vi "add 4200 initalize(SubVI).vi"(9 "字符串":string, 10 "model":string="Delta") -> (0 "连接的字符串":string, 3 "ok or cancel":bool=TRUE)   [LabVIEW 2019, in "initialize.lvlib"]
uses:
  initialize.lvlib
panel:
  in  "SMU2(Ryx) Setup":T1={"Enable"=TRUE, "Source Mode"=enum."Current Source", "Compliance (V/A)"=0.1, "Source V/I (V/A)"=0.0, "Current Measurement Range\n(Limited Auto)"=9} {"Current Measurement Range\n(Limited Auto)" items=["1 pA (pre-Amp only)", "10 pA (pre-Amp only)", "100 pA (pre-Amp only)", "1 nA", "10 nA", "100 nA", "1 uA", "10 uA", "100 uA", "1 mA", "10 mA", "100 mA", "1 A (4210-SMU only)"]; "Source V/I (V/A)" min=-100.0 max=100.0 step=0.0001 format="%^.2e"; "Compliance (V/A)" min=-210.0 max=210.0 format="%_3e"}
  in  "SMU1(Rxx) Setup":T1={"Enable"=TRUE, "Source Mode"=enum."Current Source", "Compliance (V/A)"=0.1, "Source V/I (V/A)"=0.0, "Current Measurement Range\n(Limited Auto)"=9} {"Current Measurement Range\n(Limited Auto)" items=["1 pA (pre-Amp only)", "10 pA (pre-Amp only)", "100 pA (pre-Amp only)", "1 nA", "10 nA", "100 nA", "1 uA", "10 uA", "100 uA", "1 mA", "10 mA", "100 mA", "1 A (4210-SMU only)"]; "Source V/I (V/A)" format="%^.2e"; "Compliance (V/A)" min=-210.0 max=210.0 format="%_3e"}
  in  "Integration Time":i16(slide)=2 min=1 max=3 step=1 scale=1.0..3.0
  in  "Sampling Mode Timing":T2={"Wait Time"=0.0, "Interval"=0.1, "No. of Readings"=5} {"No. of Readings" min=1 max=4097 step=1; "Interval" min=0.0 max=10.0 step=0.001 format="%.2g"; "Wait Time" min=0.0 max=100.0 step=0.1 format="%.3g"}
  out "错误输出":errorcluster
  in  "load":bool
  in  "cancel":bool
  in  "ok":bool
  # "Please make sure KI 4200 is in Normal Mode (under KCON).\nStart KXCI before running this VI."
  # "Hold up start of test (s)"
  # "Time between measurements(s)"
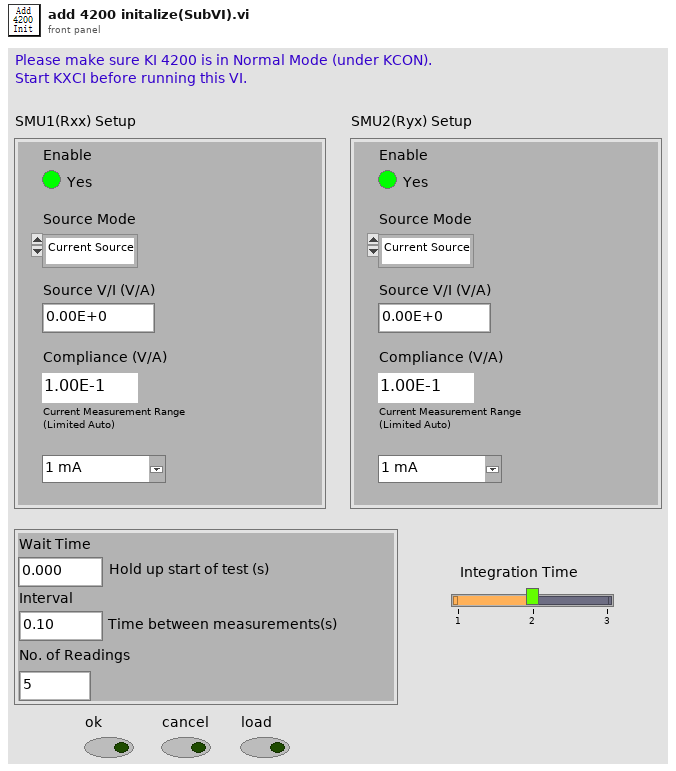
[diagram p1: front panel]
types:
  T1 = cluster{"Enable":bool, "Source Mode":enum16{"Voltage Source", "Current Source", "Common"}, "Compliance (V/A)":dbl, "Source V/I (V/A)":dbl, "Current Measurement Range\n(Limited Auto)":u16}
  T2 = cluster{"Wait Time":dbl, "Interval":dbl, "No. of Readings":i16}
  T3 = enum16{"open", "replace", "create", "open or create", "replace or create"}
  T4 = enum16{"open", "replace", "create", "open or create", "replace or create", "replace or create with confirmation"}
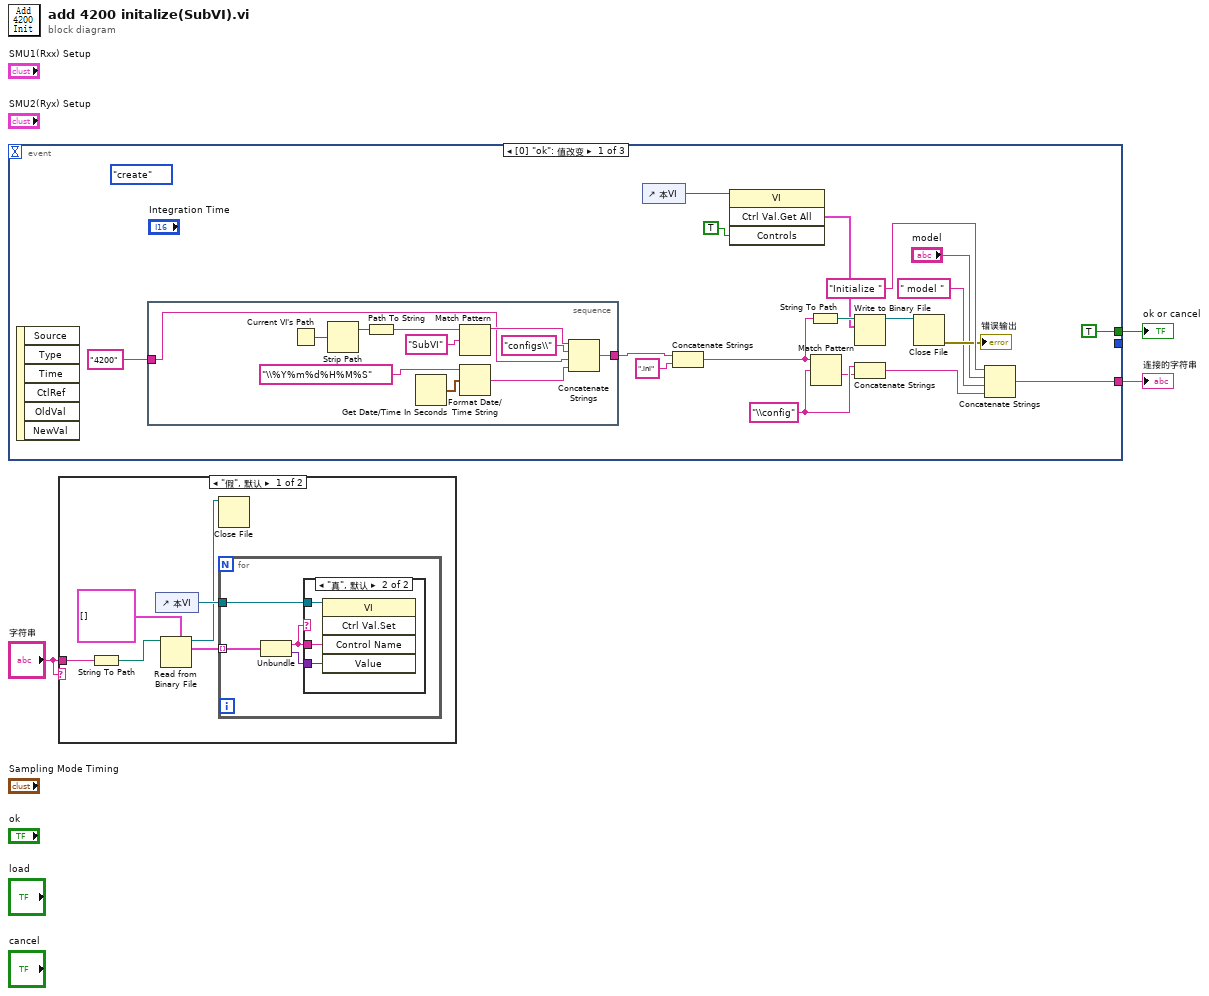
[diagram p0: block diagram]
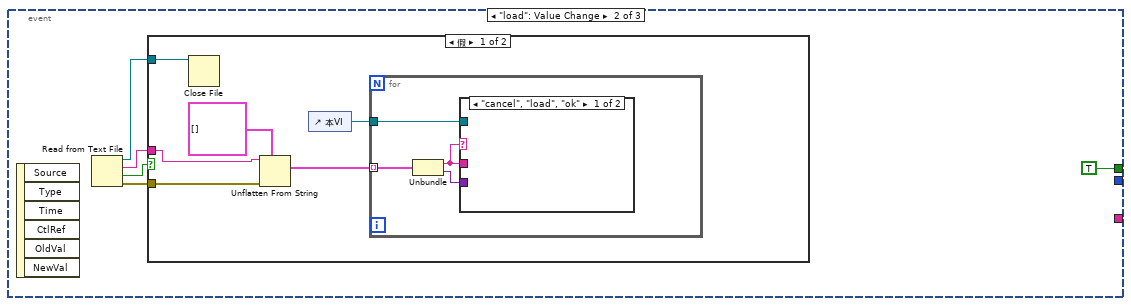
[diagram p4: hidden frame]
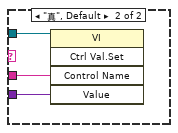
[diagram p5: hidden frame]
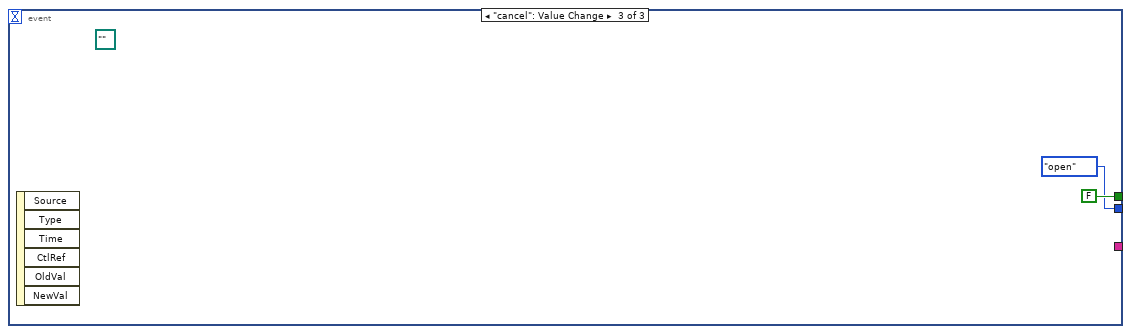
[diagram p7: hidden frame]
diagram:
  n1 = event shown="[0] \"ok\": 值改变" {
    selector: _ -> [_ _ _]
    dyn-events: _ -> [_ _ _]
    timeout: _ -> [_ _ _]
    tunnel: [_ _ T3."open" ("operation(0:open)")] -> _
    tunnel: [TRUE TRUE FALSE] -> w3
    tunnel: [w11 _ _] -> w1
    event "ok": Value Change {
      w7 = "\\config" ("正则表达式")
      (unwired) T4."create" ("操作(0:open)")
      n2 = event-data() -> ()  [unwired: 1 in, 6 out]
      n3 = stacked-sequence {
        tunnel: [w32] -> w16
        tunnel: "4200" ("字符串") -> [w22]
        frame #0 {
          n4 = Current VI's Path() -> (path=w28:path)
          n5 = Strip Path(path=w28) -> (stripped path=w23:path)  [unwired: 1 out]
          n6 = Path To String(path=w23) -> (string=w29:string)
          n7 = Get Date/Time In Seconds() -> (seconds since 1Jan1904=w26:timestamp)
          n8 = Match Pattern(string=w29, regular expression="SubVI" ("正则表达式")) -> (before substring=w31:string)  [unwired: 1 in, 3 out]
          n9 = Format Date/Time String(time format string (%c)="\\%Y%m%d%H%M%S", seconds (now)=w26) -> (date/time string=w27:string)  [unwired: 1 in]
          n10 = Concatenate Strings(w31, "configs\\" ("字符串"), w22, w27) -> (w32:string)
        }
      }
      n11 = control-ref of="本VI"() -> (w19:refnum<vi>)
      n12 = Concatenate Strings(w16, ".ini" ("字符串")) -> (w5:string)
      n13 = invoke class="VI" method="Ctrl Val.Get All"(reference=w19, "Controls"=TRUE ("控件")) -> ("Get All Control Values Variant"=w9:cluster{"Name":string, "Variant Data":variant}[])  [unwired: 2 in, 3 out]
      n14 = String To Path(string=w5) -> (path=w10:path)
      n15 = Match Pattern(string=w5, regular expression=w7) -> (after substring=w6:string)  [unwired: 1 in, 3 out]
      n16 = Write to Binary File(file (use dialog)=w10, data=w9) -> (refnum out=w8:refnum<file>)  [unwired: 4 in, 2 out]
      n17 = Concatenate Strings(w7, w6) -> (w4:string)
      n18 = Close File(refnum=w8) -> (error out=→"错误输出":errorcluster)  [unwired: 1 in, 1 out]
      n19 = Concatenate Strings("Initialize " ("字符串"), "model", " model " ("字符串"), w4) -> (w11:string)
    }
    event "load": Value Change {
      n20 = event-data() -> ()  [unwired: 1 in, 6 out]
      n21 = Read from Text File() -> (refnum out=w36:refnum<file>, text=w34:string, cancelled=w33:bool, error out=w35:errorcluster)  [unwired: 4 in]
      n22 = case shown="假" w33 {
        tunnel: w36 -> [w43 _]
        tunnel: w35 -> [w41 _]
        tunnel: w34 -> [w40 _]
        frame False {
          n23 = Close File(refnum=w43) -> ()  [unwired: 1 in, 2 out]
          n24 = Unflatten From String(type=cluster{"Name":string, "Variant Data":variant}[] [] ("控件值:获取全部"), binary string=w40, error in (no error)=w41) -> (value=w39:cluster{"Name":string, "Variant Data":variant}[])  [unwired: 2 in, 2 out]
          n25 = control-ref of="本VI"() -> (w38:refnum<vi>)
          n26 = for {
            tunnel: w39 -> [w47] mode=indexing
            tunnel: w38 -> [w46]
            n27 = Unbundle(w47) -> ("Name"=w44:string, "Variant Data"=w45:variant)
            n28 = case shown="\"cancel\", \"load\", \"ok\"" w44 {
              tunnel: w46 -> [_ w50]
              tunnel: w44 -> [_ w49]
              tunnel: w45 -> [_ w48]
              frame "cancel", "load", "ok" {
              }
              frame "真", Default {
                n29 = invoke class="VI" method="Ctrl Val.Set"(reference=w50, "Control Name"=w49, "Value"=w48) -> ()  [unwired: 2 in, 5 out]
              }
            }
          }
        }
        frame True {
        }
      }
    }
    event "cancel": Value Change {
      (unwired) path "" ("path")
      n30 = event-data() -> ()  [unwired: 1 in, 6 out]
    }
  }
  "ok or cancel" <- w3
  "连接的字符串" <- w1
  n31 = case shown="\"假\", 默认" "字符串" {
    tunnel: "字符串" -> [w58 _]
    frame "假", Default {
      n32 = String To Path(string=w58) -> (path=w56:path)
      n33 = control-ref of="本VI"() -> (w57:refnum<vi>)
      n34 = Read from Binary File(5:cluster{"Name":string, "Variant Data":variant}[] [] ("控件值:获取全部"), 11:w56) -> (2:w54:cluster{"Name":string, "Variant Data":variant}[], 3:w53:refnum<file>)  [unwired: 4 in, 2 out]
      n35 = Close File(refnum=w53) -> ()  [unwired: 1 in, 2 out]
      n36 = for {
        tunnel: w54 -> [w62] mode=indexing
        tunnel: w57 -> [w61]
        n37 = Unbundle(w62) -> ("Name"=w59:string, "Variant Data"=w60:variant)
        n38 = case shown="\"真\", 默认" w59 {
          tunnel: w61 -> [_ w65]
          tunnel: w59 -> [_ w64]
          tunnel: w60 -> [_ w63]
          frame "cancel", "load", "ok" {
          }
          frame "真", Default {
            n39 = invoke class="VI" method="Ctrl Val.Set"(reference=w65, "Control Name"=w64, "Value"=w63) -> ()  [unwired: 2 in, 5 out]
          }
        }
      }
    }
    frame "" {
    }
  }
